vi "ws DB Close.vi"(6 "Force Close? (f)":bool, 8 "error in (no error)":errorcluster, 11 "Connection Refnum":T1) -> (0 "error out":errorcluster)   [LabVIEW 2011]
uses:
  SI.LIB/ODBC/SQL Controls/Connection Refnum.ctl
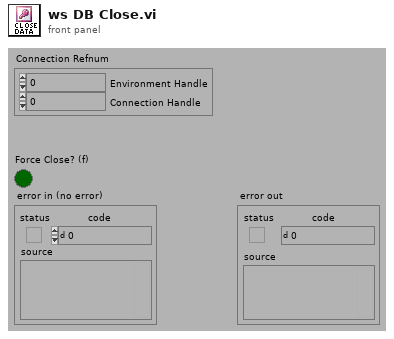
[diagram p1: front panel]
types:
  T1 = typedef "Connection Refnum.ctl" = cluster{"Environment Handle":i32, "Connection Handle":i32}
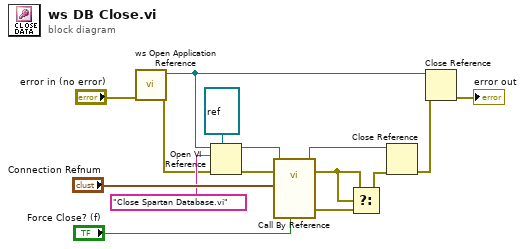
[diagram p0: block diagram]
diagram:
  n1 = call "ws Open Application Reference.vi"("error in (no error)"="error in (no error)") -> ("error out"=w2:errorcluster, "application reference"=w1:refnum<vi>)  [unwired: 9 in]
  n2 = Open VI Reference(type specifier VI Refnum (for type only)=refnum<vi> refnum, application reference (local)=w1, vi path="Close Spartan Database.vi", error in (no error)=w2) -> (vi reference=w11:refnum<vi>, error out=w12:errorcluster)  [unwired: 2 in]
  n3 = call-by-ref "?"(reference=w11, error in=w12, "Force Close? (f)"="Force Close? (f)", "Connection Refnum"="Connection Refnum") -> (reference out=w8:refnum<vi>, error out=w9:errorcluster, 0:"error out"=w10:errorcluster)  [unwired: 9 in]
  n4 = Select(t=w9, s=w9, f=w10) -> (s? t:f=w7:errorcluster)
  n5 = Close Reference(reference=w8, error in (no error)=w7) -> (error out=w6:errorcluster)
  n6 = Close Reference(reference=w1, error in (no error)=w6) -> (error out=→"error out":errorcluster)
